vi "Write Command.vi"(8 "error in (no error)":errorcluster, 10 "Command":string, 11 "UI VISA Terminal in":refnum<class "UI VISA Terminal.lvclass">) -> (0 "error out":errorcluster, 3 "UI VISA Terminal out":refnum<class "UI VISA Terminal.lvclass">)   [LabVIEW 2025, in "UI VISA Terminal.lvlib" / "UI VISA Terminal.lvclass"]
uses:
  UI VISA Terminal.lvclass
  UI VISA Terminal.lvclass/UI VISA Terminal.ctl
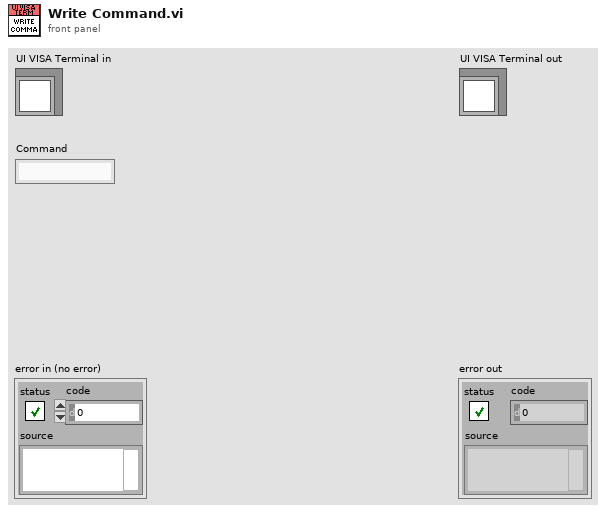
[diagram p1: front panel]
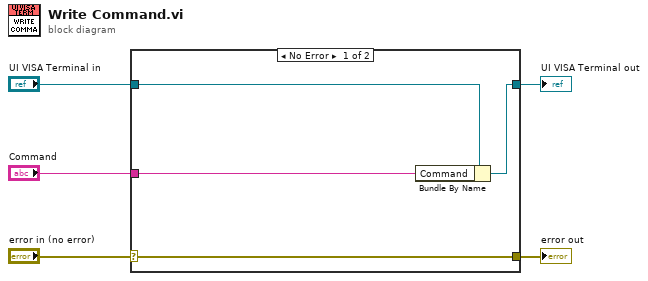
[diagram p0: block diagram]
diagram:
  n1 = case shown="No Error" "error in (no error)" {
    selector: "error in (no error)" -> [w9 w10]
    tunnel: [w9 w10] -> w4
    tunnel: [w7 w11] -> w2
    tunnel: "UI VISA Terminal in" -> [w8 w11]
    tunnel: "Command" -> [w6 _]
    frame No Error {
      n2 = Bundle By Name(cluster=w8, "Command"=w6) -> (w7:refnum<class "UI VISA Terminal.lvclass">)
    }
    frame Error {
    }
  }
  "error out" <- w4
  "UI VISA Terminal out" <- w2
